vi "Data Storage State.vi"(8 "Error In (no error)":errorcluster, 9 "Fast Data Transfer Mode (F: Off)":bool, 10 "State (0: Start)":u16(ring) items=["Start", "Pause", "Reset"], 11 "VISA Resource Name":refnum<visa-resource-name>) -> (0 "Error Out":errorcluster, 3 "VISA Resource Name Out":refnum<visa-resource-name>)   [LabVIEW 2010, in "Stanford Research 844.lvlib"]
doc: "This VI starts, pauses or resets data storage."
uses:
  <instrlib>/Stanford Research 844/Stanford Research 844.lvlib
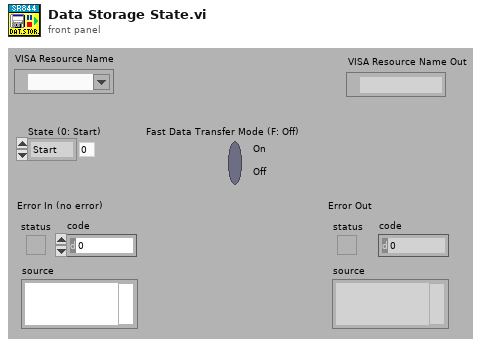
[diagram p1: front panel]
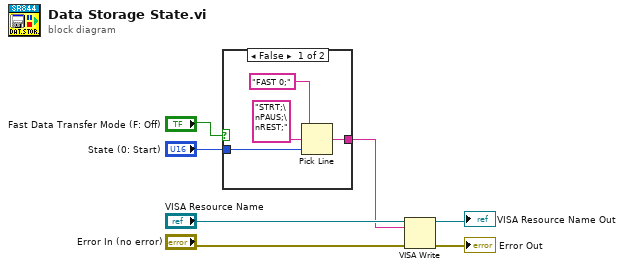
[diagram p0: block diagram]
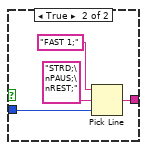
[diagram p2: hidden frame]
diagram:
  n1 = case shown="False" "Fast Data Transfer Mode (F: Off)" {
    tunnel: "State (0: Start)" -> [w11 w14]
    tunnel: [w9 w12] -> w1
    frame False {
      n2 = Pick Line(string ("")="FAST 0;", multi-line string="STRT;\nPAUS;\nREST;", line index=w11) -> (output string=w9:string)
    }
    frame True {
      n3 = Pick Line(string ("")="FAST 1;", multi-line string="STRD;\nPAUS;\nREST;", line index=w14) -> (output string=w12:string)
    }
  }
  n4 = VISA Write(VISA resource name="VISA Resource Name", write buffer=w1, error in (no error)="Error In (no error)") -> (VISA resource name out=→"VISA Resource Name Out":refnum<visa-resource-name>, error out=→"Error Out":errorcluster)  [unwired: 1 out]
